vi "set_config_cluster.vi"(8 "error in (no error)":errorcluster, 10 "config cluster variant":variant, 11 "SignalReaderCN091129DAQmx in":refnum<class "SignalReaderCN091129DAQmx.lvclass">) -> (0 "error out":errorcluster, 3 "SignalReaderCN091129DAQmx out":refnum<class "SignalReaderCN091129DAQmx.lvclass">)   [LabVIEW 2010, in "SignalReaderCN091129DAQmx.lvclass"]
uses:
  SignalReaderCN091129DAQmx.lvclass
  SignalReaderCN091129DAQmx.lvclass/SignalReaderCN091129DAQmx.ctl
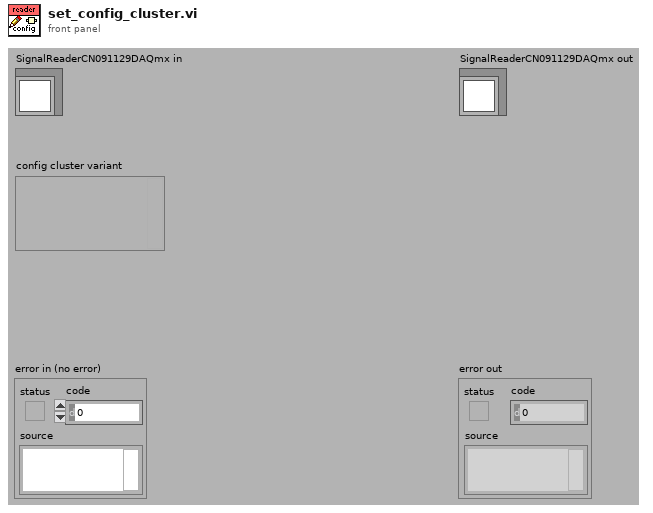
[diagram p1: front panel]
types:
  T1 = typedef "SignalReaderCN091129DAQmx.lvclass/config_data_cluster.ctl" = cluster{"analog input channels":T2[], "clock source":string, "time-out":dbl[unit], "maximum sampling rate":dbl[unit], "buffer size":i32}
  T2 = typedef "SignalReaderCN091129DAQmx.lvclass/channel_definition_cluster.ctl" = cluster{"physical Channel":string, "max_input_value":dbl, "min_input_value":dbl, "ground_reference":i32, "translation_factor":dbl, "translation_offset":dbl}
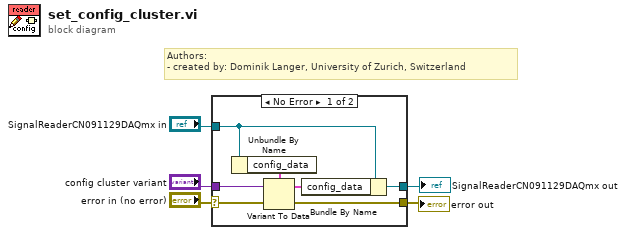
[diagram p0: block diagram]
diagram:
  # "Authors: \n- created by: Dominik Langer, University of Zurich, Switzerland"
  n1 = case shown="No Error" "error in (no error)" {
    selector: "error in (no error)" -> [w10 w13]
    tunnel: "SignalReaderCN091129DAQmx in" -> [w8 w14]
    tunnel: [w7 w13] -> w1
    tunnel: [w6 w14] -> w2
    tunnel: "config cluster variant" -> [w9 _]
    frame No Error {
      n2 = Unbundle By Name(w8) -> ("config_data"=w12:T1)
      n3 = Variant To Data(error in=w10, Variant=w9, type=w12) -> (error out=w7:errorcluster, data=w11:T1)
      n4 = Bundle By Name(cluster=w8, "config_data"=w11) -> (w6:refnum<class "SignalReaderCN091129DAQmx.lvclass">)
    }
    frame Error {
    }
  }
  "error out" <- w1
  "SignalReaderCN091129DAQmx out" <- w2
